vi "AlliGator Get Image Binning String.vi"(8 "Error In":errorcluster, 11 "Image Binning Options":T1 {"Y Bin" min=1; "X Bin" min=1}) -> (0 "Error Out":errorcluster, 3 "String":string)   [LabVIEW 2021, in "AlliGator Files.lvlib"]
doc: "Get image binning options string."
uses:
  AlliGator Image Binning Options.ctl
  AlliGator Files.lvlib
  AlliGator Source Image.lvlib
panel:
  # "see the AlliGator License on the block diagram (Ctrl+E or Window:Show Block Diagram)"
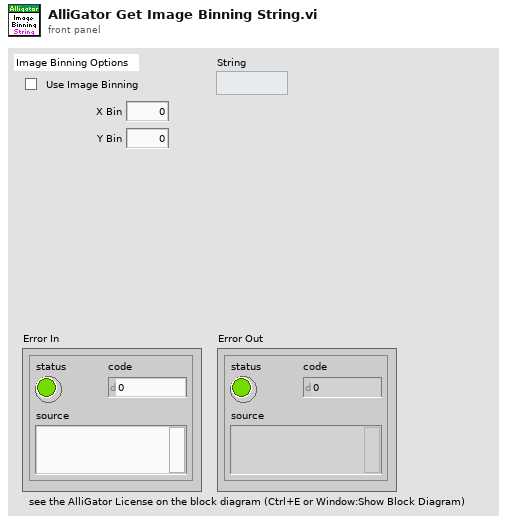
[diagram p1: front panel]
types:
  T1 = typedef "AlliGator Source Image.lvlib/AlliGator Image Binning Options.ctl" = cluster{"Use Image Binning":bool, "X Bin":i32, "Y Bin":i32}
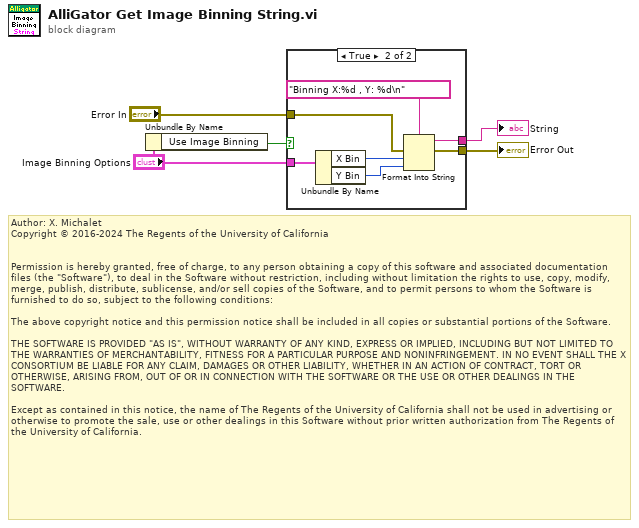
[diagram p0: block diagram]
diagram:
  # "Author: X. Michalet\nCopyright © 2016-2024 The Regents of the University of California\n \n\nPermission is hereby granted, free of charge, to any person obtaining a copy of this software and associated documentation files (the \"Software\"), to deal in the Software without restriction, including without limitation the rights to use, copy, modify, merge, publish, distribute, sublicense, and/or sell copies of the Software, and to permit persons to whom the Software is furnished to do so, subject to the following conditions:\n\nThe above copyright notice and this permission notice shall be included in all copies or substantial portions of the Software.\n\nTHE SOFTWARE IS PROVIDED \"AS IS\", WITHOUT WARRANTY OF ANY KIND, EXPRESS OR IMPLIED, INCLUDING BUT NOT LIMITED TO THE WARRANTIES OF MERCHANTABILITY, FITNESS FOR A PARTICULAR PURPOSE AND NONINFRINGEMENT. IN NO EVENT SHALL THE X CONSORTIUM BE LIABLE FOR ANY CLAIM, DAMAGES OR OTHER LIABILITY, WHETHER IN AN ACTION OF CONTRACT, TORT OR OTHERWISE, ARISING FROM, OUT OF OR IN CONNECTION WITH THE SOFTWARE OR THE USE OR OTHER DEALINGS IN THE SOFTWARE.\n\nExcept as contained in this notice, the name of The Regents of the University of California shall not be used in advertising or otherwise to promote the sale, use or other dealings in this Software without prior written authorization from The Regents of the University of California."
  n1 = Unbundle By Name("Image Binning Options") -> ("Use Image Binning"=w3:bool)
  n2 = case shown="True" w3 {
    tunnel: [_ w13] -> w5
    tunnel: "Image Binning Options" -> [_ w9]
    tunnel: "Error In" -> [w6 w12]
    tunnel: [w6 w11] -> w1
    frame False {
    }
    frame True {
      n3 = Unbundle By Name(w9) -> ("X Bin"=w8:i32, "Y Bin"=w7:i32)
      n4 = Format Into String(format string="Binning X:%d , Y: %d\n", error in=w12, w8, w7) -> (resulting string=w13:string, error out=w11:errorcluster)  [unwired: 1 in]
    }
  }
  "String" <- w5
  "Error Out" <- w1
